vi "RTS Post Voltage Frequency.vi"(0 "Chamber 1 Socket":string[][](array[string]), 1 "Chamber 2 Socket":string[][](array[string]), 2 "Chamber 3 Socket":string[][](array[string]), 3 "Chamber 4 Socket":string[][](array[string]), 5 "Error In":errorcluster, 6 "Tree Selection":T8="Select Room/Stall") -> (14 "Voltage & Freq":T1={"Voltage 1"=0.0, "Voltage 2"=0.0, "Voltage 3"=0.0, "Voltage 4"=0.0, "Voltage 5"=0.0, "Voltage 6"=0.0, "Voltage 7"=0.0, "Voltage 8"=0.0, "Frequency 1"=0, "Frequency 2"=0, "Frequency 3"=0, "Frequency 4"=0, "Frequency 5"=0, "Frequency 6"=0, "Frequency 7"=0, "Frequency 8"=0, "Ground Leak Relays"={"Ground Leakage 1"=enum."0 - Normal GL", "Ground Leakage 2"=enum."0 - Normal GL", "Ground Leakage 3"=enum."0 - Normal GL", "Ground Leakage 4"=enum."0 - Normal GL", "Ground Leakage 5"=enum."0 - Normal GL", "Ground Leakage 6"=enum."0 - Normal GL", "Ground Leakage 7"=enum."0 - Normal GL", "Ground Leakage 8"=enum."0 - Normal GL"}, "Polarity Selector"={"Station 1"=enum."Ground Neutral", "Station 2"=enum."Ground Neutral", "Station 3"=enum."Ground Neutral", "Station 4"=enum."Ground Neutral", "Station 5"=enum."Ground Neutral", "Station 6"=enum."Ground Neutral", "Station 7"=enum."Ground Neutral", "Station 8"=enum."Ground Neutral"}, "Room Setpoints"={"Room Setpoint Temperature (*RM Dry Set P1)"=90.0, "Room Setpoint Humidity (*RM Hum Set P1)"=20.0, "Room Cool Temperature (*RM Cool Setp 1)"=65.0, "Room Dehum Temperature (*RM De Hum Set P1)"=60.0}} {"Room Setpoints"."Room Dehum Temperature (*RM De Hum Set P1)" min=30.0 max=120.0; "Room Setpoints"."Room Cool Temperature (*RM Cool Setp 1)" min=30.0 max=120.0; "Room Setpoints"."Room Setpoint Humidity (*RM Hum Set P1)" min=5.0 max=98.0; "Room Setpoints"."Room Setpoint Temperature (*RM Dry Set P1)" min=40.0 max=120.0; "Frequency 8" items=["60 Hz", "50 Hz"]; "Frequency 7" items=["60 Hz", "50 Hz"]; "Frequency 6" items=["60 Hz", "50 Hz"]; "Frequency 5" items=["60 Hz", "50 Hz"]; "Frequency 4" items=["60 Hz", "50 Hz"]; "Frequency 3" items=["60 Hz", "50 Hz"]; "Frequency 2" items=["60 Hz", "50 Hz"]; "Frequency 1" items=["60 Hz", "50 Hz"]}, 19 "Error Out":errorcluster)   [LabVIEW 2020]
uses:
  Type Definitions/RTS Room Selector.ctl
  Type Definitions/RTS Voltage Frequency Settings.ctl
  Type Definitions/RTS Frequency Selector.ctl
  Drivers/WAGO 750-881/Type Definitions/Wago Ground Leakage Relays.ctl
  Drivers/WAGO 750-881/Type Definitions/Wago Ground Leakage.ctl
  Drivers/WAGO 750-881/Type Definitions/Wago Polarity Selector Relays.ctl
  Drivers/WAGO 750-881/Type Definitions/Wago Polarity Selector.ctl
  Type Definitions/RTS Chamber Temperature Humidity Control.ctl
panel:
  in  "Tab Control":enum32{"Page 1", "Page 2", "Page 3", "Page 4"}(tab)
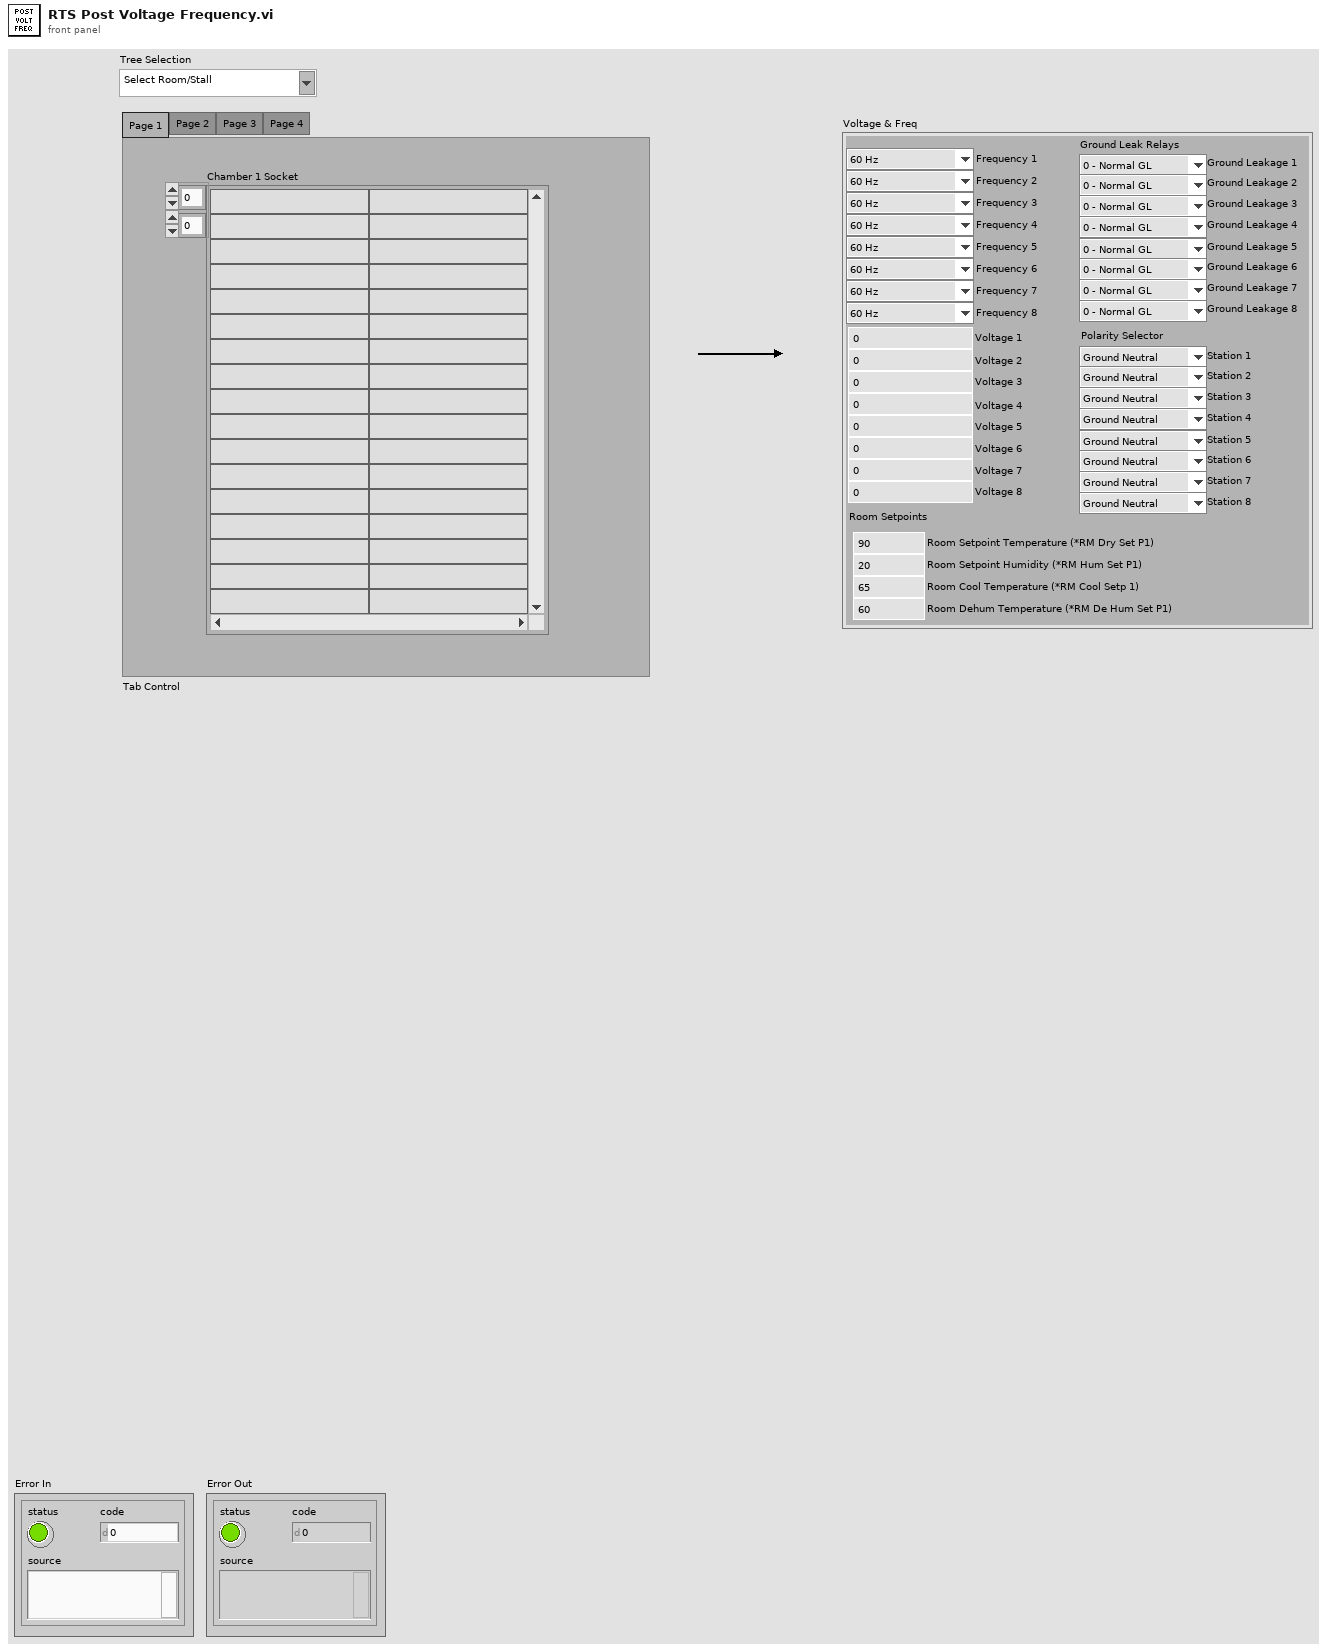
[diagram p1: front panel]
types:
  T1 = typedef "RTS Voltage Frequency Settings.ctl" = cluster{"Voltage 1":dbl, "Voltage 2":dbl, "Voltage 3":dbl, "Voltage 4":dbl, "Voltage 5":dbl, "Voltage 6":dbl, "Voltage 7":dbl, "Voltage 8":dbl, "Frequency 1":T2, "Frequency 2":T2, "Frequency 3":T2, "Frequency 4":T2, "Frequency 5":T2, "Frequency 6":T2, "Frequency 7":T2, "Frequency 8":T2, "Ground Leak Relays":T3, "Polarity Selector":T5, "Room Setpoints":T7}
  T2 = typedef "RTS Frequency Selector.ctl" = u16
  T3 = typedef "Wago Ground Leakage Relays.ctl" = cluster{"Ground Leakage 1":T4, "Ground Leakage 2":T4, "Ground Leakage 3":T4, "Ground Leakage 4":T4, "Ground Leakage 5":T4, "Ground Leakage 6":T4, "Ground Leakage 7":T4, "Ground Leakage 8":T4}
  T4 = typedef "Wago Ground Leakage.ctl" = enum16{"0 - Normal GL", "1 - Measure GL"}
  T5 = typedef "Wago Polarity Selector Relays.ctl" = cluster{"Station 1":T6, "Station 2":T6, "Station 3":T6, "Station 4":T6, "Station 5":T6, "Station 6":T6, "Station 7":T6, "Station 8":T6}
  T6 = typedef "Wago Polarity Selector.ctl" = enum16{"Ground Neutral", "Ground Line"}
  T7 = typedef "RTS Chamber Temperature Humidity Control.ctl" = cluster{"Room Setpoint Temperature (*RM Dry Set P1)":dbl, "Room Setpoint Humidity (*RM Hum Set P1)":dbl, "Room Cool Temperature (*RM Cool Setp 1)":dbl, "Room Dehum Temperature (*RM De Hum Set P1)":dbl}
  T8 = typedef "RTS Room Selector.ctl" = string
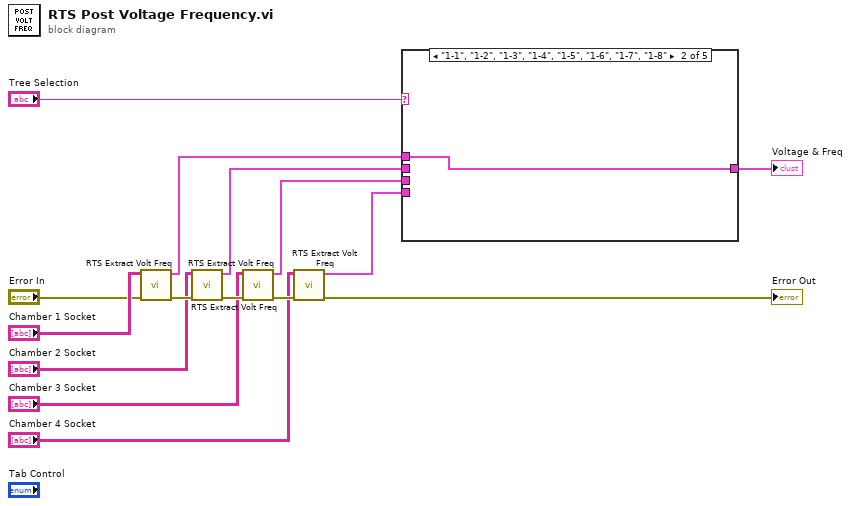
[diagram p0: block diagram]
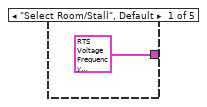
[diagram p2: hidden frame]
diagram:
  n1 = call "RTS Extract Volt Freq.vi"("Error In"="Error In", "Chamber 1 Socket"="Chamber 1 Socket") -> ("Error Out"=w14:errorcluster, "Chamber 1"=w5:T1)  [unwired: 8 in]
  n2 = call "RTS Extract Volt Freq.vi"("Error In"=w14, "Chamber 1 Socket"="Chamber 2 Socket") -> ("Error Out"=w13:errorcluster, "Chamber 1"=w4:T1)  [unwired: 8 in]
  n3 = call "RTS Extract Volt Freq.vi"("Error In"=w13, "Chamber 1 Socket"="Chamber 3 Socket") -> ("Error Out"=w12:errorcluster, "Chamber 1"=w3:T1)  [unwired: 8 in]
  n4 = call "RTS Extract Volt Freq.vi"("Error In"=w12, "Chamber 1 Socket"="Chamber 4 Socket") -> ("Error Out"=→"Error Out":errorcluster, "Chamber 1"=w2:T1)  [unwired: 8 in]
  n5 = case shown="\"1-1\", \"1-2\", \"1-3\", \"1-4\", \"1-5\", \"1-6\", \"1-7\", \"1-8\"" "Tree Selection" {
    tunnel: w5 -> [_ w17 _ _ _]
    tunnel: [T1 {"Voltage 1"=0.0, "Voltage 2"=0.0, "Voltage 3"=0.0, "Voltage 4"=0.0, "Voltage 5"=0.0, "Voltage 6"=0.0, "Voltage 7"=0.0, "Voltage 8"=0.0, "Frequency 1"=0, "Frequency 2"=0, "Frequency 3"=0, "Frequency 4"=0, "Frequency 5"=0, "Frequency 6"=0, "Frequency 7"=0, "Frequency 8"=0, "Ground Leak Relays"={"Ground Leakage 1"=enum."0 - Normal GL", "Ground Leakage 2"=enum."0 - Normal GL", "Ground Leakage 3"=enum."0 - Normal GL", "Ground Leakage 4"=enum."0 - Normal GL", "Ground Leakage 5"=enum."0 - Normal GL", "Ground Leakage 6"=enum."0 - Normal GL", "Ground Leakage 7"=enum."0 - Normal GL", "Ground Leakage 8"=enum."0 - Normal GL"}, "Polarity Selector"={"Station 1"=enum."Ground Neutral", "Station 2"=enum."Ground Neutral", "Station 3"=enum."Ground Neutral", "Station 4"=enum."Ground Neutral", "Station 5"=enum."Ground Neutral", "Station 6"=enum."Ground Neutral", "Station 7"=enum."Ground Neutral", "Station 8"=enum."Ground Neutral"}, "Room Setpoints"={"Room Setpoint Temperature (*RM Dry Set P1)"=90.0, "Room Setpoint Humidity (*RM Hum Set P1)"=20.0, "Room Cool Temperature (*RM Cool Setp 1)"=65.0, "Room Dehum Temperature (*RM De Hum Set P1)"=60.0}} ("Chamber 1") w17 w18 w19 w20] -> w1
    tunnel: w4 -> [_ _ w18 _ _]
    tunnel: w3 -> [_ _ _ w19 _]
    tunnel: w2 -> [_ _ _ _ w20]
    frame "Select Room/Stall", Default {
    }
    frame "1-1", "1-2", "1-3", "1-4", "1-5", "1-6", "1-7", "1-8" {
    }
    frame "2-1", "2-2", "2-3", "2-4", "2-5", "2-6", "2-7", "2-8" {
    }
    frame "3-1", "3-2", "3-3", "3-4", "3-5", "3-6", "3-7", "3-8" {
    }
    frame "4-1", "4-2", "4-3", "4-4", "4-5", "4-6", "4-7", "4-8" {
    }
  }
  "Voltage & Freq" <- w1
